vi "Call.vi"() -> ()   [LabVIEW 2009]
uses:
  Data/GetPixelData16.vi
  <vilib>/event_ctls.llb/eventsource.ctl
panel:
  out "Feature Name":string
  out "UsrEvtRef":refnum<user-event>
  out "Event Registration Refnum":refnum<event-registration>
  out "Event":refnum<user-event>
  out "Time":u32
  out "Type":u32
  out "Source":T1 items=["LabVIEW UI", "ActiveX", "User Event"]
  out "stop 2":bool
  out "event":bool
  out "stop":bool
  in  "Centre AOI":bool
  in  "AOI Width":i64
  in  "AOI Height":i64
  in  "error status":errorcluster
  out "Pixel Encoding":string
  out "Intensity Graph":u16[][](graph)
  out "AOIStride":i64
  in  "PreAmp":string(combo)
  out "PixelData":u16[](array[numeric])
  out "ByteData":u8[](array[numeric])
  in  "ExposureTime":dbl
  out "ImageSizeBytes":i64
  out "Handle":i32
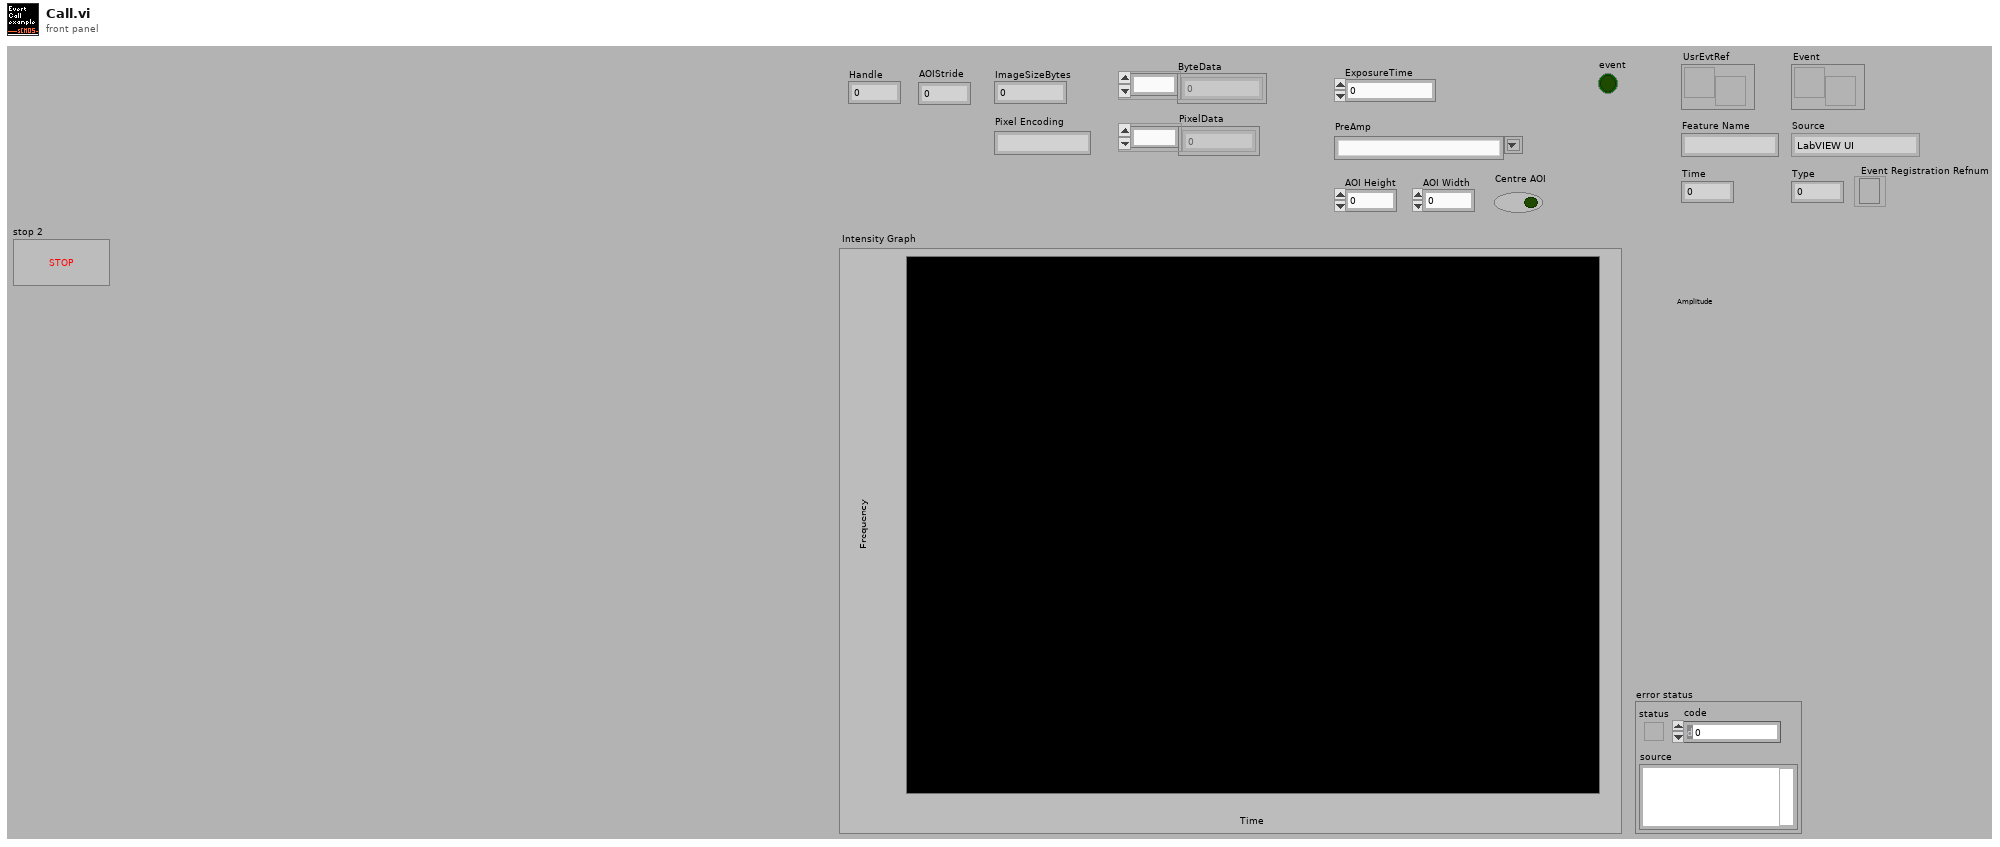
[diagram p1: front panel]
types:
  T1 = typedef "eventsource.ctl" = u32
  T2 = enum8{"Enabled", "Disabled", "Disabled and Grayed Out"}
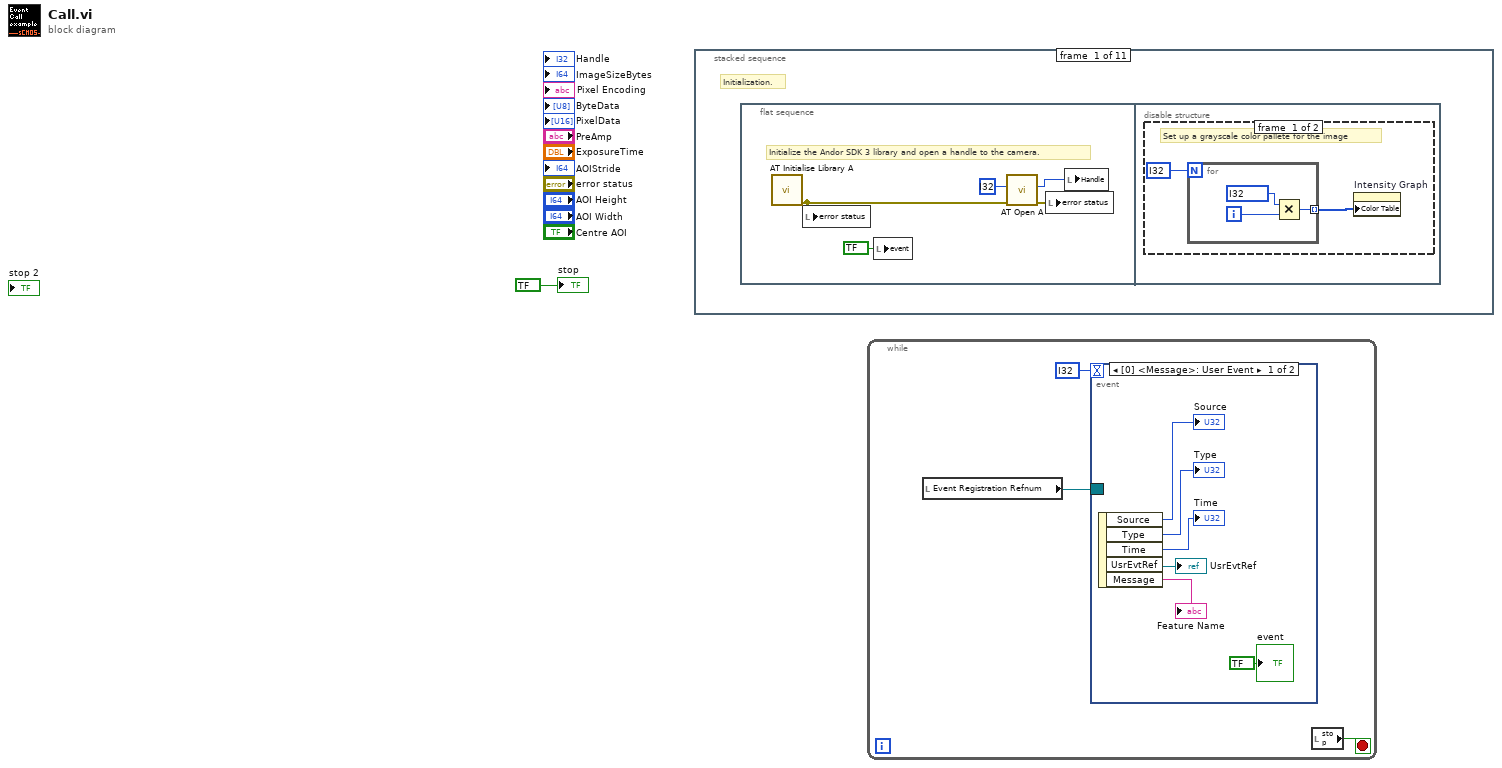
[diagram p0: block diagram]
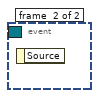
[diagram p2: hidden frame]
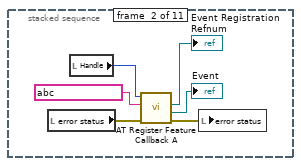
[diagram p4: hidden frame]
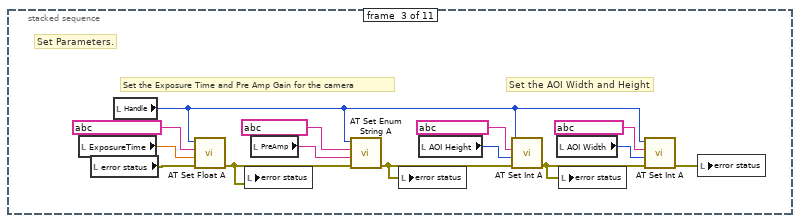
[diagram p5: hidden frame]
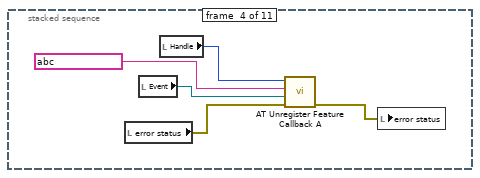
[diagram p6: hidden frame]
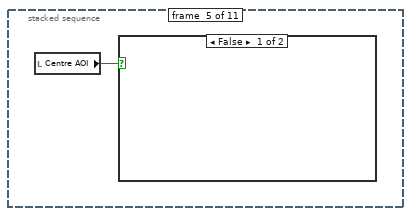
[diagram p7: hidden frame]
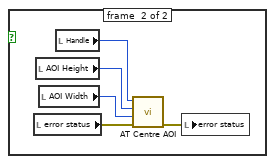
[diagram p8: hidden frame]
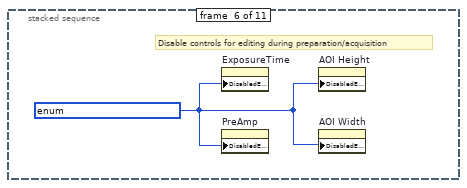
[diagram p9: hidden frame]
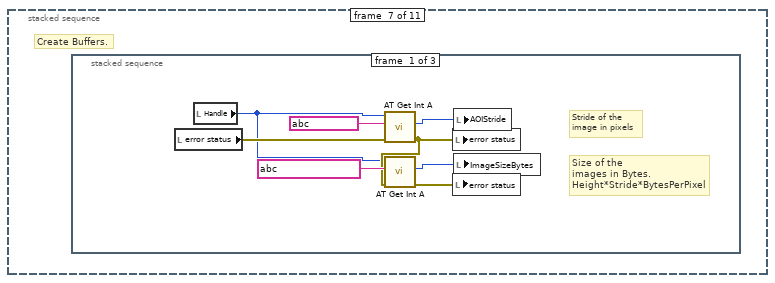
[diagram p10: hidden frame]
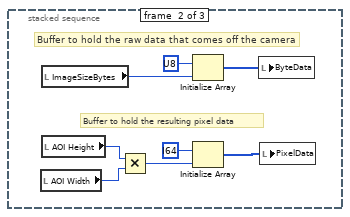
[diagram p11: hidden frame]
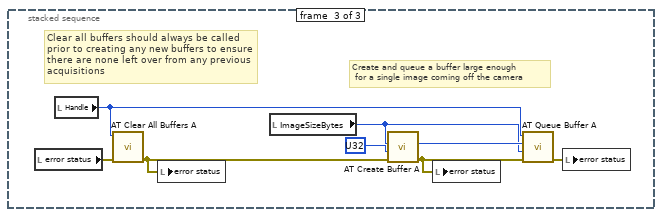
[diagram p12: hidden frame]
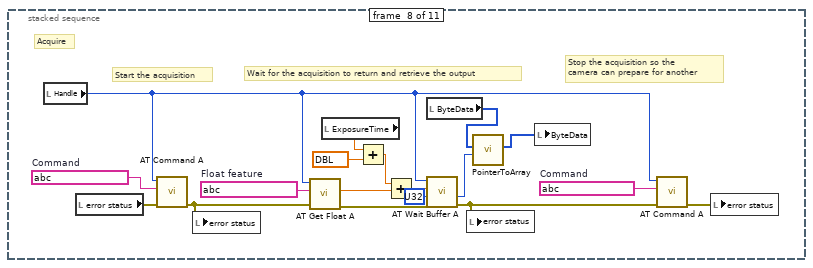
[diagram p13: hidden frame]
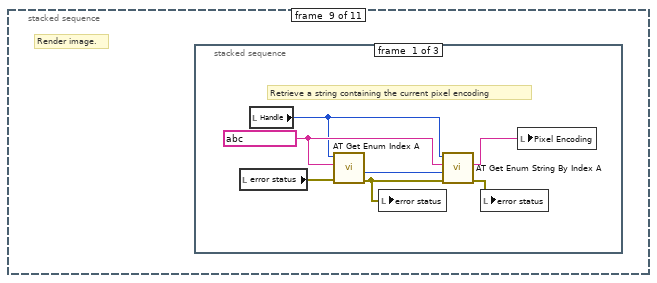
[diagram p14: hidden frame]
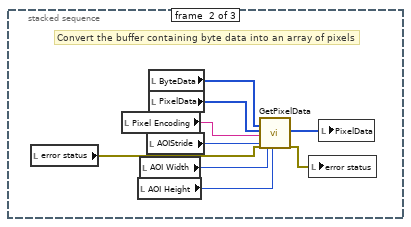
[diagram p15: hidden frame]
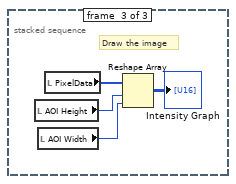
[diagram p16: hidden frame]
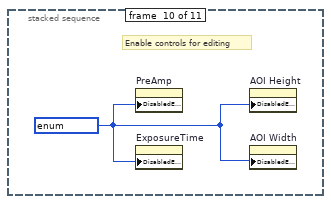
[diagram p17: hidden frame]
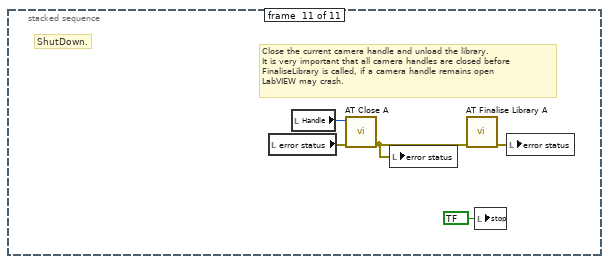
[diagram p18: hidden frame]
diagram:
  n1 = stacked-sequence {
    frame #0 {
      # "Initialization."
      n2 = flat-sequence {
        frame #0 {
          # "Initialize the Andor SDK 3 library and open a handle to the camera."
          n3 = call "AT Initialise Library A.vi"() -> ("error out"=w4:errorcluster)  [unwired: 10 in, 1 out]
          n4 = local write "error status"(w4) -> ()
          n5 = local write "event"(bool ? ("event")) -> ()
          n6 = call "AT Open A.vi"("error in (no error)"=w4, "CameraIndex"=i32 ?) -> ("error out"=w3:errorcluster, "Handle"=w5:i32)  [unwired: 7 in, 1 out]
          n7 = local write "error status"(w3) -> ()
          n8 = local write "Handle"(w5) -> ()
        }
        frame #1 {
          n9 = disable-structure shown="Enabled" {
            frame #0 {
              # "Set up a grayscale color pallete for the image"
              n10 = for {
                N: i32 ? -> [_]
                tunnel: [w10] -> w7 mode=indexing
                i -> [w11]
                n11 = Multiply(x=i32 ?, y=w11) -> (x*y=w10:i32)
              }
              n12 = property on="Intensity Graph" class="IntGraph (strict)"("Color Table"=w7) -> ()  [unwired: 2 in, 2 out]
            }
            frame #1 {
            }
          }
        }
      }
    }
    frame #1 {
      n13 = local read "error status"() -> (w14:errorcluster)
      n14 = local read "Handle"() -> (w17:i32)
      n15 = call "AT Register Feature Callback A.vi"("error in (no error)"=w14, "Feature"=string ? ("Integer feature"), "Handle"=w17) -> ("error out"=w16:errorcluster, "Event"=→"Event":refnum<user-event>, "Event Registration Refnum"=→"Event Registration Refnum":refnum<event-registration>)  [unwired: 5 in, 1 out]
      n16 = local write "error status"(w16) -> ()
    }
    frame #2 {
      # "Set the AOI Width and Height"
      # "Set the Exposure Time and Pre Amp Gain for the camera"
      # "Set Parameters."
      n17 = local read "ExposureTime"() -> (w23:dbl)
      n18 = local read "error status"() -> (w27:errorcluster)
      n19 = local read "Handle"() -> (w18:i32)
      n20 = call "AT Set Float A.vi"("error in (no error)"=w27, "Value"=w23, "Feature"=string ? ("ExposureTime"), "Hndl"=w18) -> ("error out"=w30:errorcluster)  [unwired: 6 in, 1 out]
      n21 = local write "error status"(w30) -> ()
      n22 = local read "PreAmp"() -> (w31:string)
      n23 = call "AT Set Enum String A.vi"("error in (no error)"=w30, "String"=w31, "Feature"=string ? ("SimplePreAmpGainControl"), "Handle"=w18) -> ("error out"=w26:errorcluster)  [unwired: 6 in, 1 out]
      n24 = local write "error status"(w26) -> ()
      n25 = local read "AOI Height"() -> (w20:i64)
      n26 = call "AT Set Int A.vi"("error in (no error)"=w26, "Value"=w20, "Feature"=string ? ("Integer feature 2"), "Handle"=w18) -> ("error out"=w24:errorcluster)  [unwired: 6 in, 1 out]
      n27 = local read "AOI Width"() -> (w19:i64)
      n28 = local write "error status"(w24) -> ()
      n29 = call "AT Set Int A.vi"("error in (no error)"=w24, "Value"=w19, "Feature"=string ? ("Integer feature"), "Handle"=w18) -> ("error out"=w25:errorcluster)  [unwired: 6 in, 1 out]
      n30 = local write "error status"(w25) -> ()
    }
    frame #3 {
      n31 = local read "error status"() -> (w33:errorcluster)
      n32 = local read "Event"() -> (w32:refnum<user-event>)
      n33 = local read "Handle"() -> (w36:i32)
      n34 = call "AT Unregister Feature Callback A.vi"("error in (no error)"=w33, "Event"=w32, "Feature"=string ? ("Integer feature"), "Handle"=w36) -> ("error out"=w34:errorcluster)  [unwired: 6 in, 1 out]
      n35 = local write "error status"(w34) -> ()
    }
    frame #4 {
      n36 = local read "Centre AOI"() -> (w37:bool)
      n37 = case shown="False" w37 {
        frame #0 {
        }
        frame #1 {
          n38 = local read "error status"() -> (w42:errorcluster)
          n39 = local read "AOI Height"() -> (w39:i64)
          n40 = local read "AOI Width"() -> (w38:i64)
          n41 = local read "Handle"() -> (w40:i32)
          n42 = call "AT Centre AOI.vi"("error in (no error)"=w42, "AOI Width"=w38, "AOI Height"=w39, "Handle"=w40) -> ("error out"=w41:errorcluster)  [unwired: 7 in]
          n43 = local write "error status"(w41) -> ()
        }
      }
    }
    frame #5 {
      w43 = T2 ? ("Disabled")
      # "Disable controls for editing during preparation/acquisition"
      n44 = property on="ExposureTime" class="DigNum (strict)"("DisabledEnum"=w43) -> ()  [unwired: 2 in, 2 out]
      n45 = property on="PreAmp" class="CmbBox"("DisabledEnum"=w43) -> ()  [unwired: 2 in, 2 out]
      n46 = property on="AOI Height" class="DigNum (strict)"("DisabledEnum"=w43) -> ()  [unwired: 2 in, 2 out]
      n47 = property on="AOI Width" class="DigNum (strict)"("DisabledEnum"=w43) -> ()  [unwired: 2 in, 2 out]
    }
    frame #6 {
      # "Create Buffers."
      n48 = stacked-sequence {
        frame #0 {
          # "Stride of the\nimage in pixels"
          # "Size of the\nimages in Bytes.\nHeight*Stride*BytesPerPixel"
          n49 = local read "error status"() -> (w46:errorcluster)
          n50 = local read "Handle"() -> (w44:i32)
          n51 = call "AT Get Int A.vi"("error in (no error)"=w46, "Feature"=string ? ("Integer feature"), "Handle"=w44) -> ("error out"=w47:errorcluster, "Value"=w51:i64)  [unwired: 6 in, 1 out]
          n52 = call "AT Get Int A.vi"("error in (no error)"=w47, "Feature"=string ? ("Integer feature"), "Handle"=w44) -> ("error out"=w45:errorcluster, "Value"=w50:i64)  [unwired: 6 in, 1 out]
          n53 = local write "error status"(w47) -> ()
          n54 = local write "error status"(w45) -> ()
          n55 = local write "AOIStride"(w51) -> ()
          n56 = local write "ImageSizeBytes"(w50) -> ()
        }
        frame #1 {
          # "Buffer to hold the resulting pixel data"
          # "Buffer to hold the raw data that comes off the camera"
          n57 = local read "AOI Width"() -> (w58:i64)
          n58 = local read "ImageSizeBytes"() -> (w53:i64)
          n59 = local read "AOI Height"() -> (w57:i64)
          n60 = Multiply(x=w57, y=w58) -> (x*y=w52:i64)
          n61 = Initialize Array(u8 ?, w53) -> (w55:u8[])
          n62 = Initialize Array(i64 ?, w52) -> (w56:i64[])
          n63 = local write "ByteData"(w55) -> ()
          n64 = local write "PixelData"(w56) -> ()
        }
        frame #2 {
          # "Clear all buffers should always be called \nprior to creating any new buffers to ensure\nthere are none left over from any previous \nacquisitions"
          # "Create and queue a buffer large enough\n for a single image coming off the camera"
          n65 = local read "error status"() -> (w64:errorcluster)
          n66 = local read "Handle"() -> (w60:i32)
          n67 = call "AT Clear All Buffers A.vi"("error in (no error)"=w64, "Handle"=w60) -> ("error out"=w63:errorcluster)  [unwired: 8 in, 1 out]
          n68 = local write "error status"(w63) -> ()
          n69 = local read "ImageSizeBytes"() -> (w62:i64)
          n70 = call "AT Create Buffer A.vi"("error in (no error)"=w63, "Buffer"=u32 ?, "Size"=w62) -> ("error out"=w66:errorcluster, "Buffer out"=w67:u64)  [unwired: 6 in, 1 out]
          n71 = local write "error status"(w66) -> ()
          n72 = call "AT Queue Buffer A.vi"("error in (no error)"=w66, "PtrSize"=w62, "Ptr"=w67, "Handle"=w60) -> ("error out"=w65:errorcluster)  [unwired: 6 in, 1 out]
          n73 = local write "error status"(w65) -> ()
        }
      }
    }
    frame #7 {
      w76 = string ?  # Float feature
      w79 = string ?  # Command
      w84 = string ?  # Command
      # "Stop the acquisition so the \ncamera can prepare for another"
      # "Wait for the acquisition to return and retrieve the output"
      # "Start the acquisition"
      # "Acquire"
      n74 = local read "Handle"() -> (w83:i32)
      n75 = local read "error status"() -> (w85:errorcluster)
      n76 = call "AT Command A.vi"("error in (no error)"=w85, "Feature"=w84, "Handle"=w83) -> ("error out"=w82:errorcluster)  [unwired: 7 in, 1 out]
      n77 = local write "error status"(w82) -> ()
      n78 = call "AT Get Float A.vi"("error in (no error)"=w82, "Feature"=w76, "Handle"=w83) -> ("error out"=w81:errorcluster, "Value"=w77:dbl)  [unwired: 6 in, 1 out]
      n79 = local read "ExposureTime"() -> (w75:dbl)
      n80 = Add(x=w75, y=dbl ?) -> (x+y=w73:dbl)
      n81 = Add(x=w73, y=w77) -> (x+y=w78:dbl)
      n82 = local read "ByteData"() -> (w69:u8[])
      n83 = call "AT Wait Buffer A.vi"("error in (no error)"=w81, "Input buffer"=u32 ?, "Timeout"=w78, "Handle"=w83) -> ("error out"=w71:errorcluster, "Output buffer"=w68:u64)  [unwired: 4 in, 2 out]
      n84 = local write "error status"(w71) -> ()
      n85 = call "PointerToArray.vi"("Pointer In"=w68, "Array in"=w69) -> ("Array out"=w70:u8[])  [unwired: 8 in, 1 out]
      n86 = local write "ByteData"(w70) -> ()
      n87 = call "AT Command A.vi"("error in (no error)"=w71, "Feature"=w79, "Handle"=w83) -> ("error out"=w80:errorcluster)  [unwired: 7 in, 1 out]
      n88 = local write "error status"(w80) -> ()
    }
    frame #8 {
      # "Render image."
      n89 = stacked-sequence {
        frame #0 {
          w92 = string ?
          # "Retrieve a string containing the current pixel encoding"
          n90 = local read "error status"() -> (w88:errorcluster)
          n91 = local read "Handle"() -> (w90:i32)
          n92 = call "AT Get Enum Index A.vi"("error in (no error)"=w88, "Feature"=w92, "Handle"=w90) -> ("error out"=w89:errorcluster, "Value"=w91:i32)  [unwired: 6 in, 1 out]
          n93 = local write "error status"(w89) -> ()
          n94 = call "AT Get Enum String By Index A.vi"("error in (no error)"=w89, "Index"=w91, "Feature"=w92, "Handle"=w90) -> ("error out"=w87:errorcluster, "String"=w86:string)  [unwired: 5 in, 1 out]
          n95 = local write "error status"(w87) -> ()
          n96 = local write "Pixel Encoding"(w86) -> ()
        }
        frame #1 {
          # "Convert the buffer containing byte data into an array of pixels"
          n97 = local read "error status"() -> (w94:errorcluster)
          n98 = local read "Pixel Encoding"() -> (w93:string)
          n99 = local read "AOI Height"() -> (w99:i64)
          n100 = local read "AOI Width"() -> (w100:i64)
          n101 = local read "AOIStride"() -> (w98:i64)
          n102 = local read "ByteData"() -> (w96:u8[])
          n103 = local read "PixelData"() -> (w97:u16[])
          n104 = call-poly "GetPixelData.vi"("Input buffer"=w96, "Output buffer in"=w97, "Pixel Encoding"=w93, "Stride"=w98, "error in (no error)"=w94, "Width"=w100, "Height"=w99) -> ("Output buffer out"=w101:u16[], "error out"=w95:errorcluster)  [unwired: 10 in, 1 out]
          n105 = local write "error status"(w95) -> ()
          n106 = local write "PixelData"(w101) -> ()
        }
        frame #2 {
          # "Draw the image"
          n107 = local read "AOI Height"() -> (w104:i64)
          n108 = local read "AOI Width"() -> (w103:i64)
          n109 = local read "PixelData"() -> (w105:u16[])
          n110 = Reshape Array(w105, w104, w103) -> (→"Intensity Graph":u16[][])
        }
      }
    }
    frame #9 {
      w106 = T2 ? ("Disabled")
      # "Enable controls for editing"
      n111 = property on="PreAmp" class="CmbBox"("DisabledEnum"=w106) -> ()  [unwired: 2 in, 2 out]
      n112 = property on="ExposureTime" class="DigNum (strict)"("DisabledEnum"=w106) -> ()  [unwired: 2 in, 2 out]
      n113 = property on="AOI Height" class="DigNum (strict)"("DisabledEnum"=w106) -> ()  [unwired: 2 in, 2 out]
      n114 = property on="AOI Width" class="DigNum (strict)"("DisabledEnum"=w106) -> ()  [unwired: 2 in, 2 out]
    }
    frame #10 {
      # "Close the current camera handle and unload the library.\nIt is very important that all camera handles are closed before\nFinaliseLibrary is called, if a camera handle remains open \nLabVIEW may crash."
      # "ShutDown."
      n115 = local read "error status"() -> (w110:errorcluster)
      n116 = local read "Handle"() -> (w111:i32)
      n117 = call "AT Close A.vi"("error in (no error)"=w110, "Handle"=w111) -> ("error out"=w109:errorcluster)  [unwired: 8 in, 1 out]
      n118 = local write "error status"(w109) -> ()
      n119 = call "AT Finalise Library A.vi"("error in (no error)"=w109) -> ("error out"=w108:errorcluster)  [unwired: 9 in, 1 out]
      n120 = local write "stop"(bool ? ("stop")) -> ()
      n121 = local write "error status"(w108) -> ()
    }
  }
  n122 = while {
    stop <- w114 stop-if-true
    n123 = local read "Event Registration Refnum"() -> (w112:refnum<event-registration>)
    n124 = event shown="[0] <Message>: User Event" {
      selector: w112 -> [_ _]
      dyn-events: _ -> [_ _]
      timeout: i32 ? -> [_ _]
      event #0 {
        n125 = event-data() -> ("Source"=→"Source":T1, "Type"=→"Type":u32, "Time"=→"Time":u32, "UsrEvtRef"=→"UsrEvtRef":refnum<user-event>, "Message"=→"Feature Name":string)  [unwired: 1 in]
        "event" <- bool ? ("event")
      }
      event #1 {
        n126 = event-data() -> ()  [unwired: 1 in, 1 out]
      }
    }
    n127 = local read "stop"() -> (w114:bool)
  }
  "stop" <- bool ? ("stop")
